vi "Create Arbitrary Waveform.vi"(6 "Arbitrary Numeric Waveform Data":dbl[](array[numeric])=[1000.0, 2000.0, 3000.0, 4000.0, 5000.0, 6000.0, 7000.0, 8000.0], 7 "Waveform Parameters":T1={"Frequency (1000 Hz)"=1000.0, "Amplitude (2.0 Vpp)"=2.0, "DC Offset (0.00 V)"=0.0, "Phase (0.0 degrees)"=0.002} {"Phase (0.0 degrees)" min=-360.0 max=360.0 format="%#.1g"; "DC Offset (0.00 V)" min=-10.0 max=10.0; "Amplitude (2.0 Vpp)" min=0.001 max=20.0 step=1.0 format="%#.3f"; "Frequency (1000 Hz)" min=1e-06 max=160000000.0 step=1.0 format="%#.6g"}, 8 "error in (no error)":errorcluster, 9 "Select Channel (1:Channel 1)":i32(ring)=1 items=["Channel 1"=1, "Channel 2"=2], 10 "Waveform Name (\"wave1\")":string="wave1", 11 "VISA resource name":refnum<visa-resource-name>="USB0::0xF4EC::0x1101::SDG6XEBC5R0119::INSTR") -> (0 "error out":errorcluster, 3 "VISA resource name out":refnum<visa-resource-name>)   [LabVIEW 2018, in "SDG X Series.lvlib"]
doc: "Creates and saves an arbitrary (user-defined) waveform in non-volatile memory, then selects it for output."
uses:
  SDG X Series/SDG X Series.lvlib
panel:
  # "Will upload file, change to arb wavefunction with the uploaded waveform\nselected"
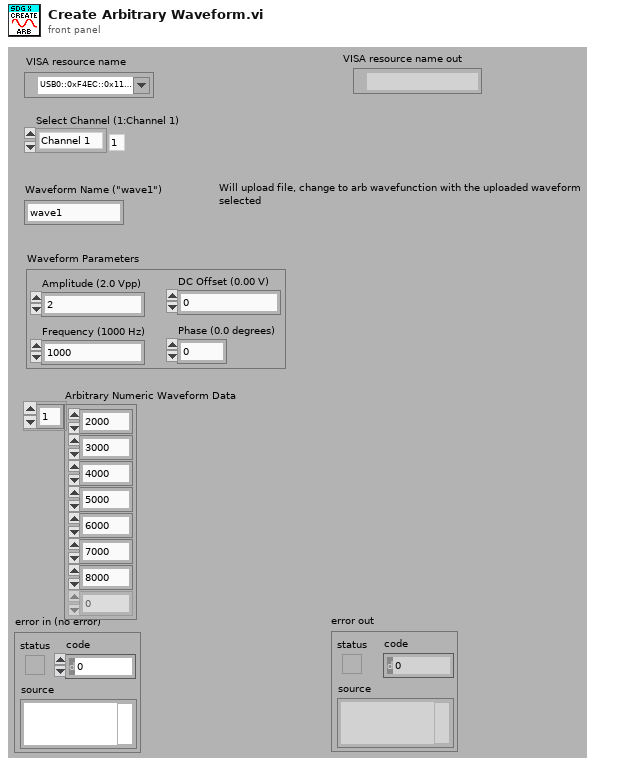
[diagram p1: front panel]
types:
  T1 = cluster{"Frequency (1000 Hz)":dbl, "Amplitude (2.0 Vpp)":dbl, "DC Offset (0.00 V)":dbl, "Phase (0.0 degrees)":dbl}
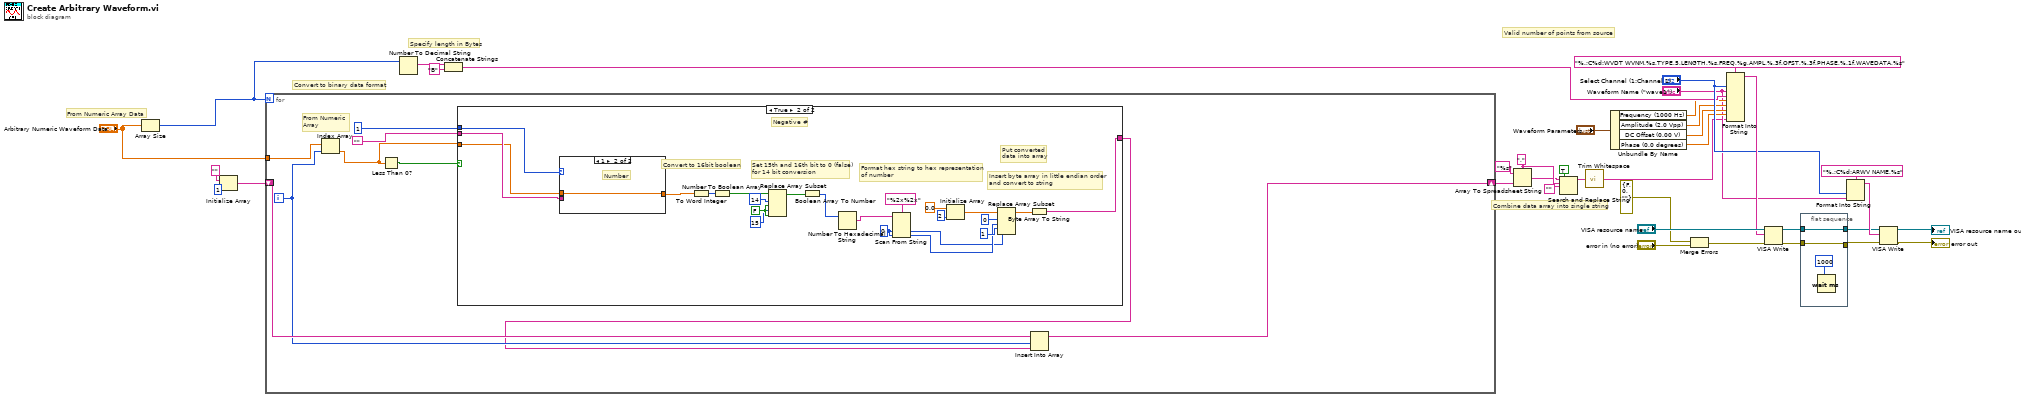
[diagram p0: block diagram]
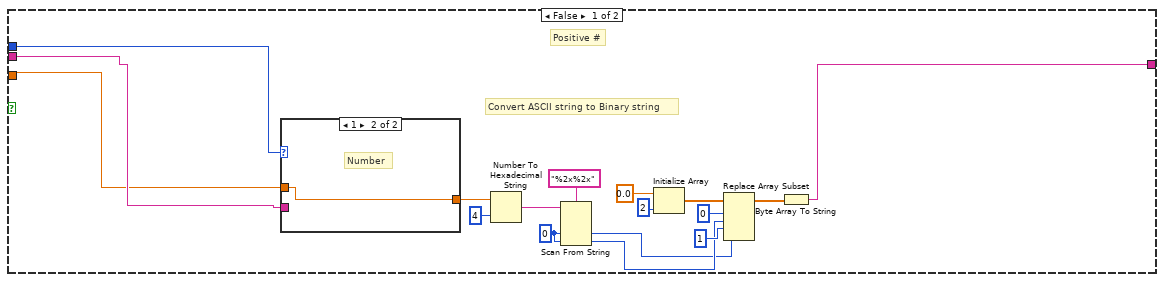
[diagram p2: hidden frame]
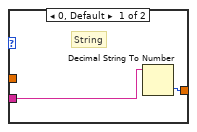
[diagram p3: hidden frame]
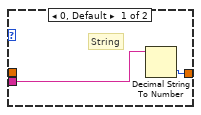
[diagram p4: hidden frame]
diagram:
  w22 = ","
  # "From Numeric Array Data"
  # "Specify length in Bytes"
  # "Combine data array into single string"
  # "Valid number of points from source"
  # "Convert to binary data format"
  n1 = Array Size(array="Arbitrary Numeric Waveform Data") -> (size(s)=w30:i32)
  n2 = Initialize Array("", 1) -> (w26:string[])
  n3 = for {
    N: w30 -> [_]
    tunnel: "Arbitrary Numeric Waveform Data" -> [w42]
    shift-right: [w38] -> w7
    shift-left: w26 -> [w41]
    i -> [w40]
    # "From Numeric\nArray"
    # "Put converted\ndata into array"
    n4 = Index Array(array=w42, index=w40) -> (element=w45:dbl)
    n5 = Less Than 0?(x=w45) -> (x < 0?=w46:bool)
    n6 = case shown="True" w46 {
      tunnel: w45 -> [w47 w67]
      tunnel: [w48 w68] -> w39
      tunnel: "" -> [w49 w69]
      tunnel: u16 1 -> [w50 w70]
      frame False {
        w59 = 0 ("default value 1")
        # "Convert ASCII string to Binary string"
        # "Positive #"
        n7 = case shown="1" w50 {
          tunnel: [w65 w66] -> w60
          tunnel: w49 -> [w64 _]
          tunnel: w47 -> [_ w66]
          frame 0, Default {
            # "String"
            n8 = Decimal String To Number(string=w64) -> (number=w65:i32)  [unwired: 2 in, 1 out]
          }
          frame 1 {
            # "Number"
          }
        }
        n9 = Number To Hexadecimal String(1:i16 4 ("width (-)"), 2:w60) -> (0:w62:string)
        n10 = Scan From String(format string="%2x%2x", input string=w62, default 1=w59, default 2=w59) -> (output 1=w51:i32, output 2=w52:i32)  [unwired: 2 in, 3 out]
        n11 = Initialize Array(0.0 ("element"), 2) -> (w57:dbl[])
        n12 = Replace Array Subset(array=w57, new element #1=w52, index #1=0, new element #2=w51, index #2=1) -> (w54:dbl[])
        n13 = Byte Array To String(unsigned byte array=w54) -> (string=w48:string)
      }
      frame True {
        w81 = 0 ("default value 1")
        w88 = FALSE
        # "Insert byte array in little endian order\nand convert to string"
        # "Format hex string to hex representation\nof number"
        # "Set 15th and 16th bit to 0 (false)\nfor 14 bit conversion"
        # "Convert to 16bit boolean"
        # "Negative #"
        n14 = case shown="1" w70 {
          tunnel: [w91 w92] -> w71
          tunnel: w69 -> [w90 _]
          tunnel: w67 -> [_ w92]
          frame 0, Default {
            # "String"
            n15 = Decimal String To Number(string=w90) -> (number=w91:i32)  [unwired: 2 in, 1 out]
          }
          frame 1 {
            # "Number"
          }
        }
        n16 = To Word Integer(number=w71) -> (16bit integer=w89:i16)
        n17 = Number To Boolean Array(number=w89) -> (Boolean array=w85:bool[])
        n18 = Replace Array Subset(array=w85, new element #1=w88, index #1=14, new element #2=w88, index #2=15) -> (w84:bool[])
        n19 = Boolean Array To Number(Boolean array=w84) -> (number=w83:u32)
        n20 = Number To Hexadecimal String(2:w83) -> (0:w72:string)  [unwired: 1 in]
        n21 = Scan From String(format string="%2x%2x", input string=w72, default 1=w81, default 2=w81) -> (output 1=w73:i32, output 2=w74:i32)  [unwired: 2 in, 3 out]
        n22 = Initialize Array(0.0 ("element"), 2) -> (w79:dbl[])
        n23 = Replace Array Subset(array=w79, new element #1=w74, index #1=0, new element #2=w73, index #2=1) -> (w76:dbl[])
        n24 = Byte Array To String(unsigned byte array=w76) -> (string=w68:string)
      }
    }
    n25 = Insert Into Array(array=w41, index=w40, new element=w39) -> (w38:string[])
  }
  n26 = Number To Decimal String(number=w30) -> (decimal integer string=w16:string)  [unwired: 1 in]
  n27 = Concatenate Strings(w16, "B" ("string")) -> (w14:string)
  n28 = Array To Spreadsheet String(delimiter (Tab)=w22, array=w7, 3:"%s") -> (spreadsheet string=w19:string)
  n29 = Search and Replace String(replace all?=TRUE, input string=w19, search string=w22, replace string="") -> (result string=w20:string)  [unwired: 4 in, 3 out]
  n30 = call <vilib>:"Trim Whitespace.vi"("string"=w20) -> ("trimmed string"=w8:string)  [unwired: 1 in]
  n31 = Unbundle By Name("Waveform Parameters") -> ("Frequency (1000 Hz)"=w13:dbl, "Amplitude (2.0 Vpp)"=w12:dbl, "DC Offset (0.00 V)"=w11:dbl, "Phase (0.0 degrees)"=w10:dbl)
  n32 = Merge Errors(errorcluster {"status"=FALSE, "code"=0, "source"=""} ("error constant"), "error in (no error)") -> (w32:errorcluster)
  n33 = Format Into String(format string="%.;C%d:WVDT WVNM,%s,TYPE,5,LENGTH,%s,FREQ,%g,AMPL,%.3f,OFST,%.3f,PHASE,%.1f,WAVEDATA,%s", "Select Channel (1:Channel 1)", "Waveform Name (\"wave1\")", w14, w13, w12, w11, w10, w8) -> (resulting string=w35:string)  [unwired: 2 in, 1 out]
  n34 = VISA Write(VISA resource name="VISA resource name", write buffer=w35, error in (no error)=w32) -> (VISA resource name out=w4:refnum<visa-resource-name>, error out=w3:errorcluster)  [unwired: 1 out]
  n35 = flat-sequence {
    tunnel: w4 -> [w94]
    tunnel: w3 -> [w93]
    tunnel: [w94] -> w2
    tunnel: [w93] -> w1
    frame #0 {
      n36 = Wait (ms)(milliseconds to wait=1000 ("x")) -> ()  [unwired: 1 out]
    }
  }
  n37 = Format Into String(format string="%.;C%d:ARWV NAME,%s", "Select Channel (1:Channel 1)", "Waveform Name (\"wave1\")") -> (resulting string=w31:string)  [unwired: 2 in, 1 out]
  n38 = VISA Write(VISA resource name=w2, write buffer=w31, error in (no error)=w1) -> (VISA resource name out=→"VISA resource name out":refnum<visa-resource-name>, error out=→"error out":errorcluster)  [unwired: 1 out]
